vi "ColoredNoiseGeneration_example.vi"() -> ()   [LabVIEW 2015]
uses:
  <vilib>/Analysis/1siggen.llb/Ramp Pattern by Samples.vi
  <vilib>/Analysis/2dsp.llb/Inverse Real FFT.vi
  <vilib>/measure/maresamp.llb/Resample Pair of Arrays (single shot).vi
  <vilib>/Analysis/NI_AALBase.lvlib
  <vilib>/gmath/NI_Gmath.lvlib
  <vilib>/Analysis/NI_AALPro.lvlib
  <vilib>/measure/NI_MAPro.lvlib
panel:
  in  "Fs (Hz)":dbl=1000.0 format="%#_13g"
  in  "number of points":i32=20000
  in  "Frequency Envelope":cluster{"frequency":dbl, "noise density":dbl}[](array[cluster])=[{"frequency"=0.0, "noise density"=0.8999999999999999}, {"frequency"=5.0, "noise density"=0.8}, {"frequency"=10.0, "noise density"=0.7}, {"frequency"=50.0, "noise density"=0.5}, {"frequency"=100.0, "noise density"=0.4}, {"frequency"=500.0, "noise density"=0.0}] {"noise density" min=0.0 step=0.1}
  out "Noise density":cluster{"f0":dbl, "df":dbl, "magnitude":dbl[]}[](graph)
  out "Colored Noise Signal":waveform(dbl)(graph)
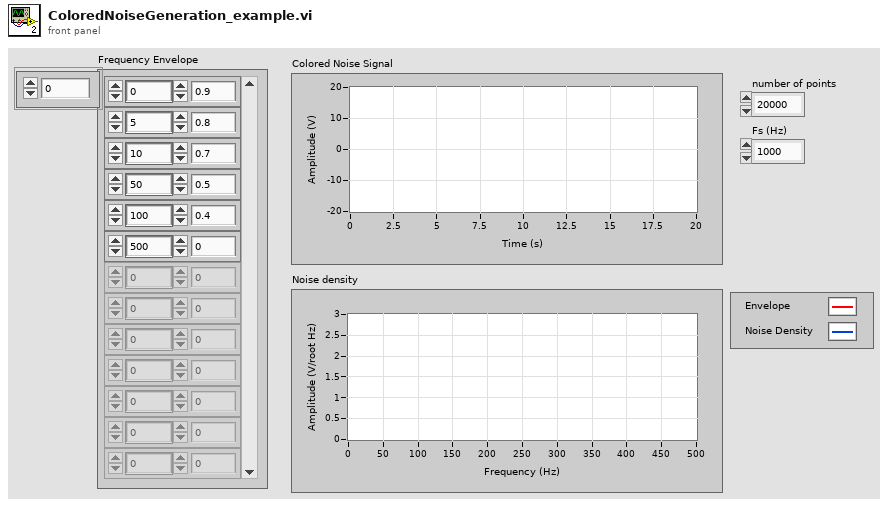
[diagram p1: front panel]
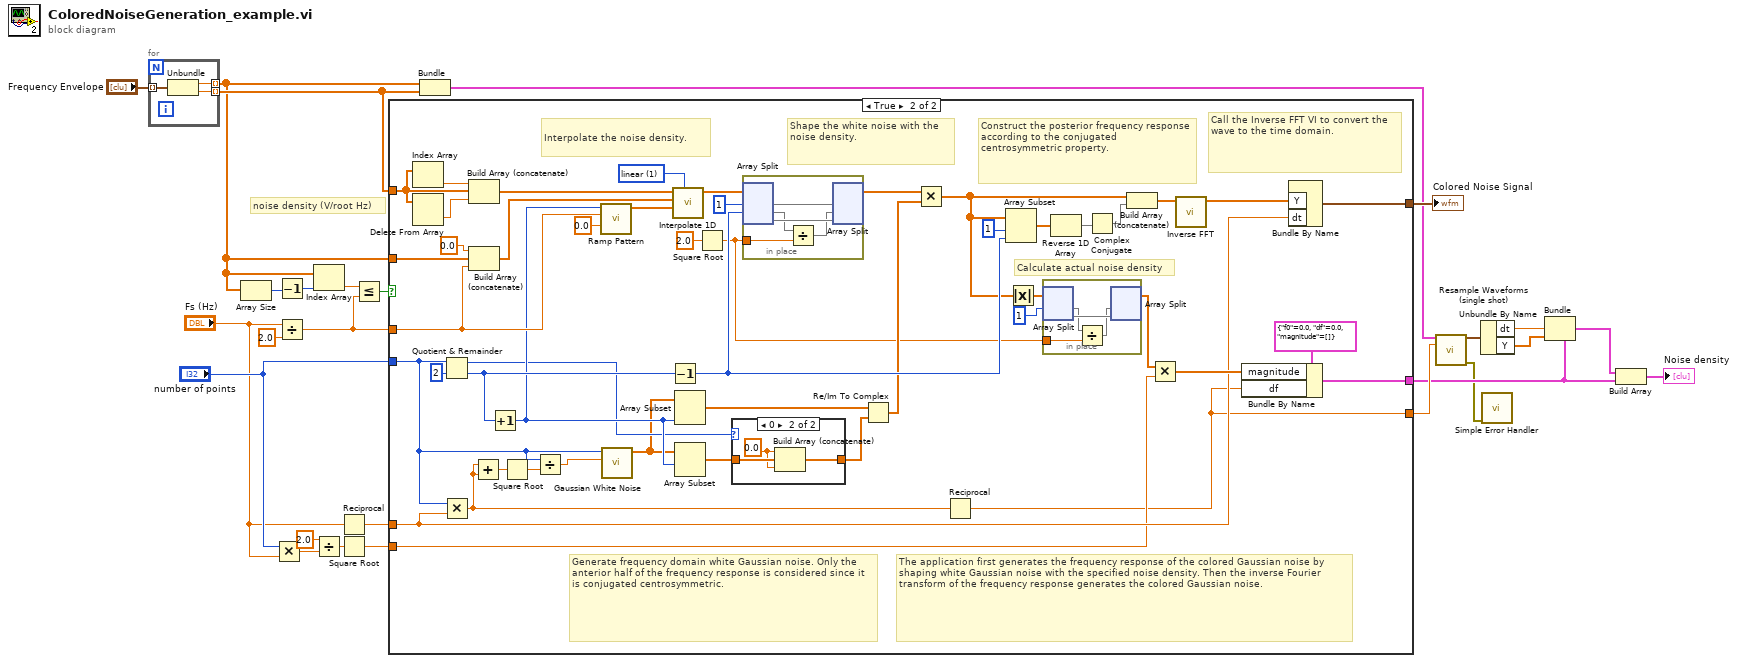
[diagram p0: block diagram]
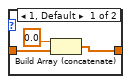
[diagram p3: hidden frame]
diagram:
  # "noise density (V/root Hz)"
  n1 = for {
    tunnel: "Frequency Envelope" -> [w29] mode=indexing
    tunnel: [w28] -> w2 mode=indexing
    tunnel: [w27] -> w3 mode=indexing
    n2 = Unbundle(w29) -> ("frequency"=w28:dbl, "noise density"=w27:dbl)
  }
  n3 = Array Size(array=w2) -> (size(s)=w24:i32)
  n4 = Multiply(x="number of points", y="Fs (Hz)") -> (x*y=w17:dbl)
  n5 = Decrement(x=w24) -> (x-1=w23:i32)
  n6 = Divide(x="Fs (Hz)", y=2.0) -> (x/y=w21:dbl)
  n7 = Index Array(array=w2, index=w23) -> (element=w25:dbl)
  n8 = Divide(x=2.0, y=w17) -> (x/y=w15:dbl)
  n9 = Reciprocal(x="Fs (Hz)") -> (1/x=w20:dbl)
  n10 = Square Root(x=w15) -> (sqrt(x)=w14:dbl)
  n11 = Less Or Equal?(x=w25, y=w21) -> (x <= y?=w22:bool)
  n12 = case shown="True" w22 {
    tunnel: w3 -> [_ w48]
    tunnel: "number of points" -> [_ w34]
    tunnel: [_ w60] -> w13
    tunnel: w21 -> [_ w67]
    tunnel: w2 -> [_ w69]
    tunnel: w20 -> [_ w37]
    tunnel: [_ w40] -> w7
    tunnel: w14 -> [_ w31]
    tunnel: [_ w30] -> w11
    frame False {
    }
    frame True {
      w71 = 1 items=["nearest", "linear", "spline", "cubic Hermite", "Lagrange"] ("method")
      # "The application first generates the frequency response of the colored Gaussian noise by shaping white Gaussian noise with the specified noise density. Then the inverse Fourier transform of the frequency response generates the colored Gaussian noise."
      # "Calculate actual noise density"
      # "Construct the posterior frequency response according to the conjugated centrosymmetric property."
      # "Generate frequency domain white Gaussian noise. Only the anterior half of the frequency response is considered since it is conjugated centrosymmetric."
      # "Call the Inverse FFT VI to convert the wave to the time domain."
      # "Shape the white noise with the noise density."
      # "Interpolate the noise density."
      n13 = Index Array(array=w48) -> (element=w59:dbl)  [unwired: 1 in]
      n14 = Delete From Array(array=w48) -> (deleted portion=w47:dbl)  [unwired: 2 in, 1 out]
      n15 = Quotient & Remainder(x=w34, y=2) -> (x-y*floor(x/y)=w55:i32, floor(x/y)=w66:i32)
      n16 = Multiply(x=w34, y=w37) -> (x*y=w44:dbl)
      n17 = Build Array (concatenate)(w59, w48, w47) -> (w70:dbl[])
      n18 = Build Array (concatenate) "Build Array"(0.0, w69, w67) -> (w68:dbl[])
      n19 = Add(x=w44, y=w44) -> (x+y=w56:dbl)
      n20 = Increment(x=w66) -> (x+1=w58:i32)
      n21 = Square Root(x=w56) -> (sqrt(x)=w61:dbl)
      n22 = Divide(x=w34, y=w61) -> (x/y=w33:dbl)
      n23 = call-poly <vilib>:"Ramp Pattern.vi"("start"=0.0, "end"=w67, "samples"=w58) -> ("Ramp Pattern"=w76:dbl[])  [unwired: 7 in, 1 out]
      n24 = call <vilib>:"Gaussian White Noise.vi"("standard deviation"=w33, "samples"=w34) -> ("Gaussian noise pattern"=w32:dbl[])  [unwired: 8 in, 1 out]
      n25 = Decrement(x=w66) -> (x-1=w64:i32)
      n26 = call <vilib>:"Interpolate 1D.vi"("method"=w71, "xi"=w76, "X"=w68, "Y"=w70) -> ("yi"=w50:dbl[])  [unwired: 5 in, 2 out]
      n27 = Array Subset(array=w32, length=w58) -> (w54:dbl[])  [unwired: 1 in]
      n28 = Array Subset(array=w32, index=w58) -> (w74:dbl[])  [unwired: 1 in]
      n29 = Square Root(x=2.0) -> (sqrt(x)=w35:dbl)
      n30 = case shown="0" w55 {
        tunnel: w74 -> [w84 w87]
        tunnel: [w82 w85] -> w53
        frame 1, Default {
          n31 = Build Array (concatenate)(0.0, w84) -> (w82:dbl[])
        }
        frame 0 {
          w86 = 0.0
          n32 = Build Array (concatenate)(w86, w87, w86) -> (w85:dbl[])
        }
      }
      n33 = in-place {
        in-place-border: w35 -> [w88]
        n34 = in-place-split #1(w50, 1, w64) -> (w92:dbl[], w90:dbl[], w91:dbl[])
        n35 = Divide(x=w90, y=w88) -> (x/y=w89:dbl[])
        n36 = in-place-split #1(w92, w89, w91) -> (w62:dbl[])  [unwired: 2 out]
      }
      n37 = Re/Im To Complex(1:w53, 2:w54) -> (0:w52:cdb[])
      n38 = Multiply(x=w62, y=w52) -> (x*y=w42:cdb[])
      n39 = Reciprocal(x=w44) -> (1/x=w30:dbl)
      n40 = Array Subset(array=w42, index=1, length=w64) -> (w72:cdb[])
      n41 = Absolute Value(x=w42) -> (abs(x)=w43:dbl[])
      n42 = in-place {
        in-place-border: w35 -> [w78]
        n43 = in-place-split #2(w43, 1) -> (w79:dbl[], w81:dbl[])
        n44 = Divide(x=w79, y=w78) -> (x/y=w80:dbl[])
        n45 = in-place-split #2(w80, w81) -> (w39:dbl[])  [unwired: 1 out]
      }
      n46 = Reverse 1D Array(array=w72) -> (reversed array=w46:cdb[])
      n47 = Complex Conjugate(1:w46) -> (0:w45:cdb[])
      n48 = Build Array (concatenate)(w42, w45) -> (w51:cdb[])
      n49 = Multiply(x=w39, y=w31) -> (x*y=w38:dbl[])
      n50 = call-poly <vilib>:"Inverse FFT.vi"("FFT {X}"=w51) -> ("X"=w57:dbl[])  [unwired: 9 in, 1 out]
      n51 = Bundle By Name(cluster=cluster{"f0":dbl, "df":dbl, "magnitude":dbl[]} {"f0"=0.0, "df"=0.0, "magnitude"=[]} ("PSD"), "magnitude"=w38, "df"=w30) -> (w40:cluster{"f0":dbl, "df":dbl, "magnitude":dbl[]})
      n52 = Bundle By Name("Y"=w57, "dt"=w37) -> (w60:waveform(dbl))  [unwired: 1 in]
    }
  }
  "Colored Noise Signal" <- w13
  n53 = Bundle(w2, w3) -> (w12:cluster{dbl[], dbl[]})  [unwired: 1 in]
  n54 = call-poly <vilib>:"Resample Waveforms (single shot).vi"("XY-data in"=w12, "dt"=w11) -> ("resampled waveform out"=w10:waveform(dbl), "error out"=w1:errorcluster)  [unwired: 9 in, 3 out]
  n55 = Unbundle By Name(w10) -> ("dt"=w9:dbl, "Y"=w8:dbl[])
  n56 = call <vilib>:"Simple Error Handler.vi"("error in (no error)"=w1) -> ()  [unwired: 4 in, 5 out]
  n57 = Bundle(cluster=w7, "df"=w9, "magnitude"=w8) -> (w6:cluster{"f0":dbl, "df":dbl, "magnitude":dbl[]})  [unwired: 1 in]
  n58 = Build Array(w6, w7) -> (→"Noise density":cluster{"f0":dbl, "df":dbl, "magnitude":dbl[]}[])
